vi "Notifier & Queue.vi"() -> ()   [LabVIEW 2020]
panel:
  out "Waveform Chart 2":dbl(graph)
  out "Waveform Chart":dbl(graph)
  # "Notifier"
  # "Queue"
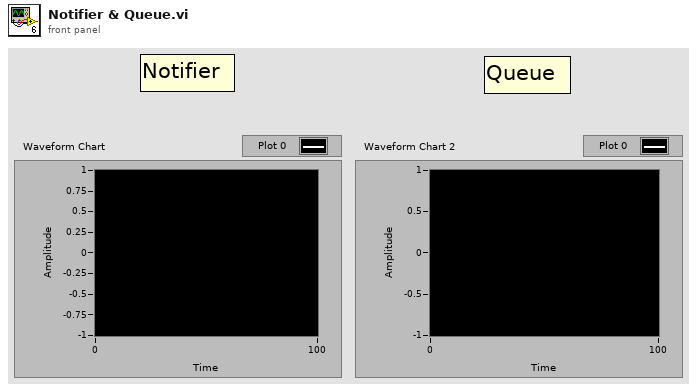
[diagram p1: front panel]
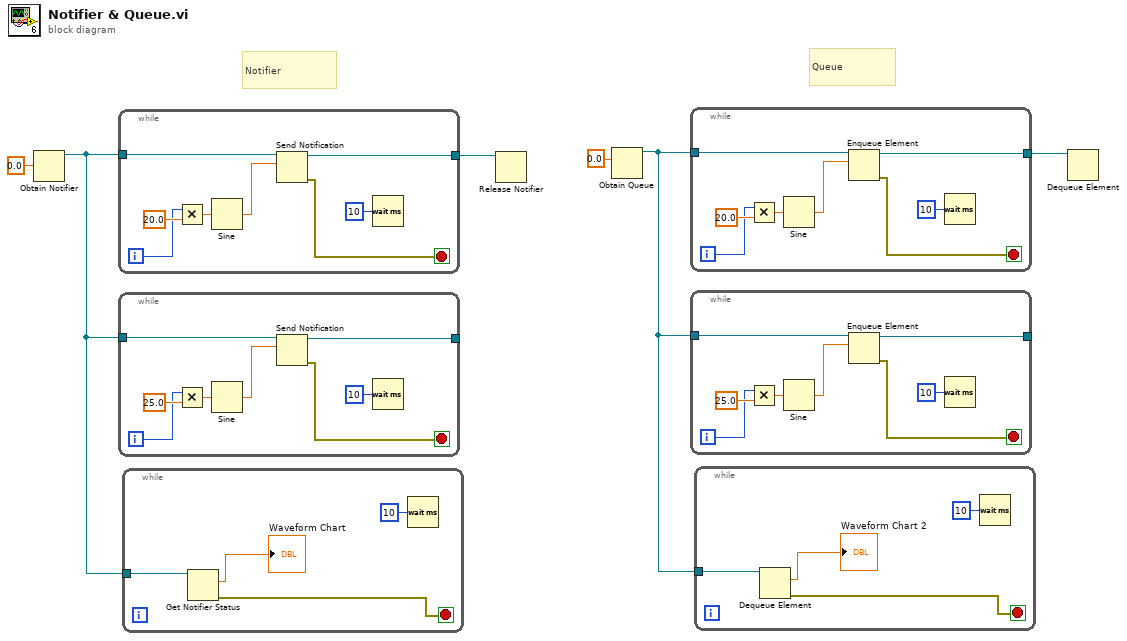
[diagram p0: block diagram]
diagram:
  # "Queue"
  # "Notifier"
  n1 = Obtain Notifier(notification data type=0.0) -> (notifier out=w4:refnum<notifier>)  [unwired: 3 in, 2 out]
  n2 = while {
    tunnel: w4 -> [w14]
    tunnel: [w13] -> w6
    i -> [w9]
    stop <- w11 stop-if-true
    n3 = Multiply(x=w9, y=20.0) -> (x*y=w12:dbl)
    n4 = Sine(x=w12) -> (sin(x)=w7:dbl)
    n5 = Send Notification(notification=w7, notifier=w14) -> (notifier out=w13:refnum<notifier>, error out=w11:errorcluster)  [unwired: 1 in]
    n6 = Wait (ms)(milliseconds to wait=u32 10) -> ()  [unwired: 1 out]
  }
  n7 = while {
    tunnel: w4 -> [w22]
    tunnel: [w21] -> _
    i -> [w17]
    stop <- w19 stop-if-true
    n8 = Multiply(x=w17, y=25.0) -> (x*y=w20:dbl)
    n9 = Sine(x=w20) -> (sin(x)=w15:dbl)
    n10 = Send Notification(notification=w15, notifier=w22) -> (notifier out=w21:refnum<notifier>, error out=w19:errorcluster)  [unwired: 1 in]
    n11 = Wait (ms)(milliseconds to wait=u32 10) -> ()  [unwired: 1 out]
  }
  n12 = while {
    tunnel: w4 -> [w25]
    stop <- w24 stop-if-true
    n13 = Get Notifier Status(notifier=w25) -> (current notification=→"Waveform Chart":dbl, error out=w24:errorcluster)  [unwired: 1 in, 3 out]
    n14 = Wait (ms)(milliseconds to wait=u32 10) -> ()  [unwired: 1 out]
  }
  n15 = Release Notifier(notifier=w6) -> ()  [unwired: 2 in, 3 out]
  n16 = Obtain Queue(element data type=0.0) -> (queue out=w1:refnum<queue>)  [unwired: 4 in, 2 out]
  n17 = while {
    tunnel: w1 -> [w34]
    tunnel: [w33] -> w3
    i -> [w29]
    stop <- w31 stop-if-true
    n18 = Multiply(x=w29, y=20.0) -> (x*y=w32:dbl)
    n19 = Sine(x=w32) -> (sin(x)=w27:dbl)
    n20 = Enqueue Element(queue=w34, element=w27) -> (queue out=w33:refnum<queue>, error out=w31:errorcluster)  [unwired: 2 in, 1 out]
    n21 = Wait (ms)(milliseconds to wait=u32 10) -> ()  [unwired: 1 out]
  }
  n22 = while {
    tunnel: w1 -> [w42]
    tunnel: [w41] -> _
    i -> [w37]
    stop <- w39 stop-if-true
    n23 = Multiply(x=w37, y=25.0) -> (x*y=w40:dbl)
    n24 = Sine(x=w40) -> (sin(x)=w35:dbl)
    n25 = Enqueue Element(queue=w42, element=w35) -> (queue out=w41:refnum<queue>, error out=w39:errorcluster)  [unwired: 2 in, 1 out]
    n26 = Wait (ms)(milliseconds to wait=u32 10) -> ()  [unwired: 1 out]
  }
  n27 = while {
    tunnel: w1 -> [w45]
    stop <- w44 stop-if-true
    n28 = Dequeue Element(queue=w45) -> (element=→"Waveform Chart 2":dbl, error out=w44:errorcluster)  [unwired: 2 in, 2 out]
    n29 = Wait (ms)(milliseconds to wait=u32 10) -> ()  [unwired: 1 out]
  }
  n30 = Dequeue Element(queue=w3) -> ()  [unwired: 2 in, 4 out]
